vi "oax_Sync DSA and TIO (DAQmx DSA).vi"(4 "Slave Slot Number":i32(ring) caption="PXI Slot Number" items=["Slot 3", "Slot 4", "Slot 5", "Slot 6", "Slot 7", "Slot 8", "Slot 9", "Slot 10", "Slot 11", "Slot 12", "Slot 13", "Slot 14", "Slot 15", "Slot 16"], 6 "DSA device type":T1 items=["4472"=0, "4474"=10, "4461"=1, "4462"=11, "4464"=12, "449x"=6, "9232"=7, "9233"=2, "9234"=3, "9229"=4, "9239"=5], 8 "error in":errorcluster, 10 "TIO task in":refnum<k21>, 11 "DSA task in":refnum<k21>) -> (0 "error out":errorcluster, 2 "TIO task out":refnum<k21>, 3 "DSA task out":refnum<k21>)   [LabVIEW 2017]
uses:
  <vilib>/addons/Sound and Vibration/Order Analysis/Example Support/sub VIs/OAXML_DSA Device Type.ctl
  <resource>/objmgr/daqmx.rc
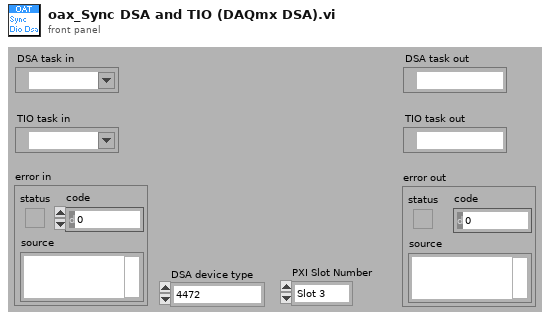
[diagram p1: front panel]
types:
  T1 = typedef "OAXML_DSA Device Type.ctl" = u16
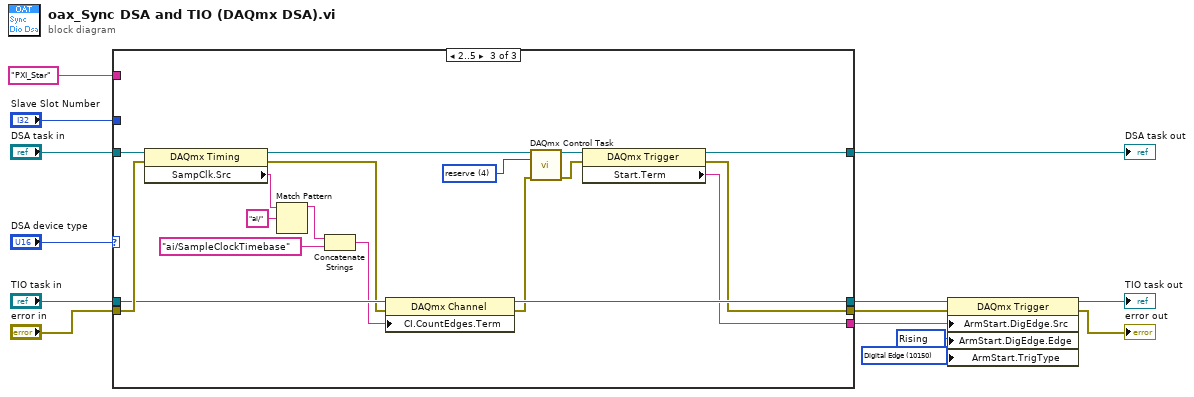
[diagram p0: block diagram]
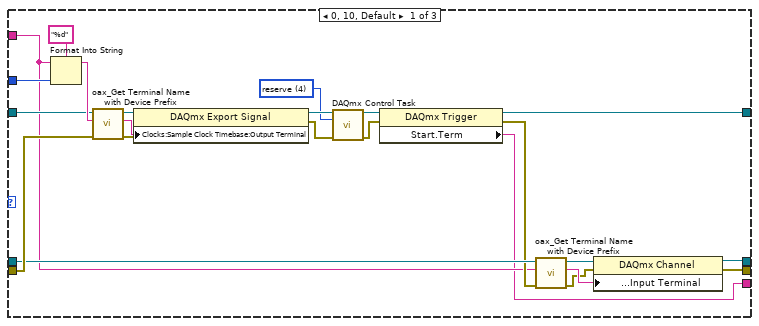
[diagram p2: hidden frame]
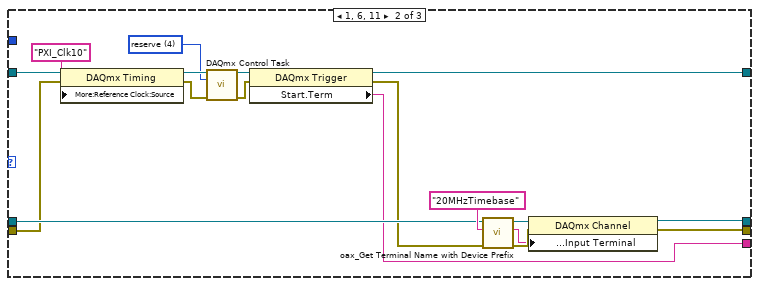
[diagram p3: hidden frame]
diagram:
  w6 = 10150 items=["Digital Edge"=10150, "None"=10230] ("ArmStart.TrigType")
  w7 = 10280 items=["Rising"=10280, "Falling"=10171] ("ArmStart.DigEdge.Edge")
  n1 = case shown="2..5" "DSA device type" {
    tunnel: [w25 w45 w64] -> w14
    tunnel: "DSA task in" -> [w29 w53 w73]
    tunnel: "TIO task in" -> [w26 w49 w71]
    tunnel: [w30 w48 w62] -> w2
    tunnel: [w31 w47 w63] -> w4
    tunnel: "error in" -> [w28 w46 w72]
    tunnel: "Slave Slot Number" -> [w27 _ _]
    tunnel: "PXI_Star" ("Local Terminal Name") -> [w23 _ _]
    tunnel: [w22 w43 w61] -> w5
    frame 0, 10, Default {
      w15 = 4 items=["verify"=2, "reserve"=4, "commit"=3, "unreserve"=5, "abort"=6] ("action")
      n2 = Format Into String(format string="%d", initial string=w23, w27) -> (resulting string=w33:string)  [unwired: 1 in, 1 out]
      n3 = call <vilib>:"oax_Get Terminal Name with Device Prefix.vi"("error in (no error)"=w28, "Local Terminal Name"=w33, "task/channels in"=w29) -> ("error out"=w35:errorcluster, "Terminal Name with Device Prefix"=w34:tag, "task out"=w36:refnum<k21>)  [unwired: 6 in]
      n4 = property class="DAQmx Export Signal"(reference=w36, error in=w35, "Clocks:Sample Clock Timebase:Output Terminal"=w34) -> (reference out=w17:refnum<k21>, error out=w19:errorcluster)
      n5 = call <vilib>:"DAQmx Control Task.vi"("task/channels in"=w17, "action"=w15, "error in"=w19) -> ("task out"=w16:refnum<k21>, "error out"=w18:errorcluster)  [unwired: 11 in]
      n6 = property class="DAQmx Trigger"(reference=w16, error in=w18) -> (reference out=w25:refnum<k21>, error out=w24:errorcluster, "Start.Term"=w22:tag)
      n7 = call <vilib>:"oax_Get Terminal Name with Device Prefix.vi"("error in (no error)"=w24, "Local Terminal Name"=w23, "task/channels in"=w26) -> ("error out"=w20:errorcluster, "Terminal Name with Device Prefix"=w21:tag, "task out"=w32:refnum<k21>)  [unwired: 6 in]
      n8 = property class="DAQmx Channel"(reference=w32, error in=w20, "Counter Input:Count Edges:Input Terminal"=w21) -> (reference out=w31:refnum<k21>, error out=w30:errorcluster)
    }
    frame 1, 6, 11 {
      w38 = 4 items=["verify"=2, "reserve"=4, "commit"=3, "unreserve"=5, "abort"=6] ("action")
      n9 = property class="DAQmx Timing"(reference=w53, error in=w46, "More:Reference Clock:Source"="PXI_Clk10" ("Local Terminal Name")) -> (reference out=w42:refnum<k21>, error out=w40:errorcluster)
      n10 = call <vilib>:"DAQmx Control Task.vi"("task/channels in"=w42, "action"=w38, "error in"=w40) -> ("task out"=w41:refnum<k21>, "error out"=w39:errorcluster)  [unwired: 11 in]
      n11 = property class="DAQmx Trigger"(reference=w41, error in=w39) -> (reference out=w45:refnum<k21>, error out=w44:errorcluster, "Start.Term"=w43:tag)
      n12 = call <vilib>:"oax_Get Terminal Name with Device Prefix.vi"("error in (no error)"=w44, "Local Terminal Name"="20MHzTimebase", "task/channels in"=w49) -> ("error out"=w52:errorcluster, "Terminal Name with Device Prefix"=w51:tag, "task out"=w50:refnum<k21>)  [unwired: 6 in]
      n13 = property class="DAQmx Channel"(reference=w50, error in=w52, "Counter Input:Count Edges:Input Terminal"=w51) -> (reference out=w47:refnum<k21>, error out=w48:errorcluster)
    }
    frame 2..5 {
      w56 = 4 items=["verify"=2, "reserve"=4, "commit"=3, "unreserve"=5, "abort"=6] ("action")
      n14 = property class="DAQmx Timing"(reference=w73, error in=w72) -> (reference out=w60:refnum<k21>, error out=w70:errorcluster, "SampClk.Src"=w69:tag)
      n15 = Match Pattern(string=w69, regular expression="ai/") -> (before substring=w67:string)  [unwired: 1 in, 3 out]
      n16 = Concatenate Strings(w67, "ai/SampleClockTimebase" ("string")) -> (w65:string)
      n17 = property class="DAQmx Channel"(reference=w71, error in=w70, "CI.CountEdges.Term"=w65) -> (reference out=w63:refnum<k21>, error out=w58:errorcluster)
      n18 = call <vilib>:"DAQmx Control Task.vi"("task/channels in"=w60, "action"=w56, "error in"=w58) -> ("task out"=w59:refnum<k21>, "error out"=w57:errorcluster)  [unwired: 11 in]
      n19 = property class="DAQmx Trigger"(reference=w59, error in=w57) -> (reference out=w64:refnum<k21>, error out=w62:errorcluster, "Start.Term"=w61:tag)
    }
  }
  "DSA task out" <- w14
  n20 = property class="DAQmx Trigger"(reference=w4, error in=w2, "ArmStart.DigEdge.Src"=w5, "ArmStart.DigEdge.Edge"=w7, "ArmStart.TrigType"=w6) -> (reference out=→"TIO task out":refnum<k21>, error out=→"error out":errorcluster)
